vi "Config PM Step Increment.vi"(0 "VISA Resource Name":refnum<visa-resource-name>, 1 "Internal Frequency (0: UP)":i16(ring) items=["UP", "DOWN"], 2 "Frequency Step (1.0)":dbl=1.0, 5 "Path (0:1)":enum16{"1", "2"}(ring), 7 "Deviation  (0: UP)":i16(ring) items=["UP", "DOWN"], 9 "Deviation Step (1.0)":dbl=1.0, 11 "error in (no error)":errorcluster {"code" format="%.0x"}) -> (4 "VISA Resource Name Out":refnum<visa-resource-name>, 15 "error out":errorcluster {"code" format="%.0x"})   [LabVIEW 2014, in "Agilent ESG Series.lvlib"]
doc: "This VI configures PM Step Increment parameters.\n\nNotes:\n(1) This VI is supported for Agilent E4438C only."
uses:
  Agilent ESG Series.lvlib
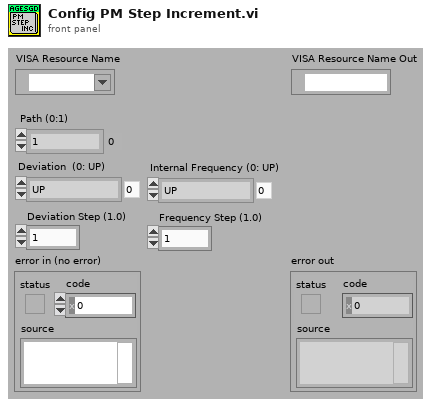
[diagram p1: front panel]
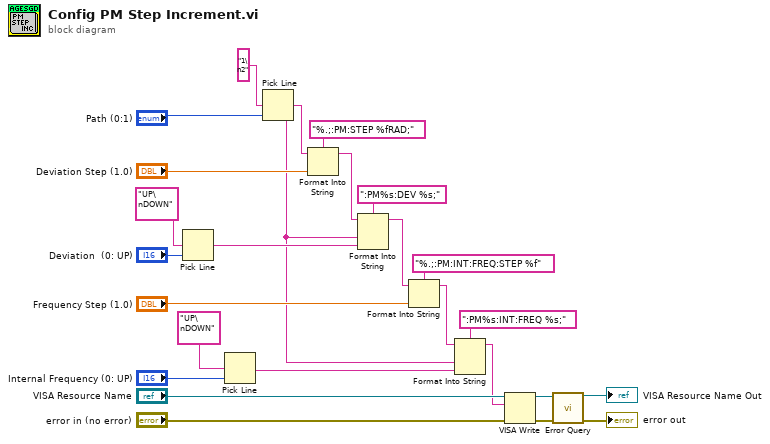
[diagram p0: block diagram]
diagram:
  n1 = Pick Line(multi-line string="UP\nDOWN", line index="Deviation  (0: UP)") -> (output string=w13:string)  [unwired: 1 in]
  n2 = Pick Line(multi-line string="UP\nDOWN", line index="Internal Frequency (0: UP)") -> (output string=w16:string)  [unwired: 1 in]
  n3 = Pick Line(multi-line string="1\n2", line index="Path (0:1)") -> (output string=w4:string)  [unwired: 1 in]
  n4 = Format Into String(format string="%.;:PM:STEP %fRAD;", initial string=w4, "Deviation Step (1.0)") -> (resulting string=w5:string)  [unwired: 1 in, 1 out]
  n5 = Format Into String(format string=":PM%s:DEV %s;", initial string=w5, w4, w13) -> (resulting string=w3:string)  [unwired: 1 in, 1 out]
  n6 = Format Into String(format string="%.;:PM:INT:FREQ:STEP %f", initial string=w3, "Frequency Step (1.0)") -> (resulting string=w2:string)  [unwired: 1 in, 1 out]
  n7 = Format Into String(format string=":PM%s:INT:FREQ %s;", initial string=w2, w4, w16) -> (resulting string=w1:string)  [unwired: 1 in, 1 out]
  n8 = VISA Write(VISA resource name="VISA Resource Name", write buffer=w1, error in (no error)="error in (no error)") -> (VISA resource name out=w21:refnum<visa-resource-name>, error out=w20:errorcluster)  [unwired: 1 out]
  n9 = call "Error Query.vi"("VISA Resource Name"=w21, "error in (no error)"=w20) -> ("VISA Resource Name Out"=→"VISA Resource Name Out":refnum<visa-resource-name>, "error out"=→"error out":errorcluster)  [unwired: 10 in, 2 out]
